vi "仪器连通测试VI.vi"(4 "断开通讯":bool, 7 "motor link":bool, 8 "error in (no error)":errorcluster caption="错误输入（无错误）", 9 "rotation num":dbl, 10 "target position":dbl=0.2 min=0.2 max=25.0 step=0.002) -> (0 "error out":errorcluster caption="错误输出", 1 "rotaion":dbl, 2 "position":dbl)   [LabVIEW 2017]
doc: "该模板用于创建子VI。"
uses:
  motor control.ctl
panel:
  in  "DaisyChain settings for rotation":T1={"Register DC"=FALSE, "DaisyChain Search?"=TRUE, "Device ID"=1}
  in  "USB settings for rotation":cluster{"S/N":string, "USB Search?":bool}={"S/N"="0135500392", "USB Search?"=FALSE}
  in  "System no. 2":i32=1 min=1 step=1
  in  "DaisyChain setting for move":T1={"Register DC"=FALSE, "DaisyChain Search?"=TRUE, "Device ID"=1}
  in  "USB setting for move":cluster{"S/N":string, "USB Search?":bool}={"S/N"="0135500392", "USB Search?"=FALSE}
  in  "minimal rot error":dbl=0.001
  in  "minimal error":dbl=0.001
  in  "motor control":T2={"System no."=1, "Conn. \nAxes"=[], "当前数值"=[]} {"System no." min=1 step=1}
  in  "System no.":i32=1 min=1 step=1
  # "parameter set"
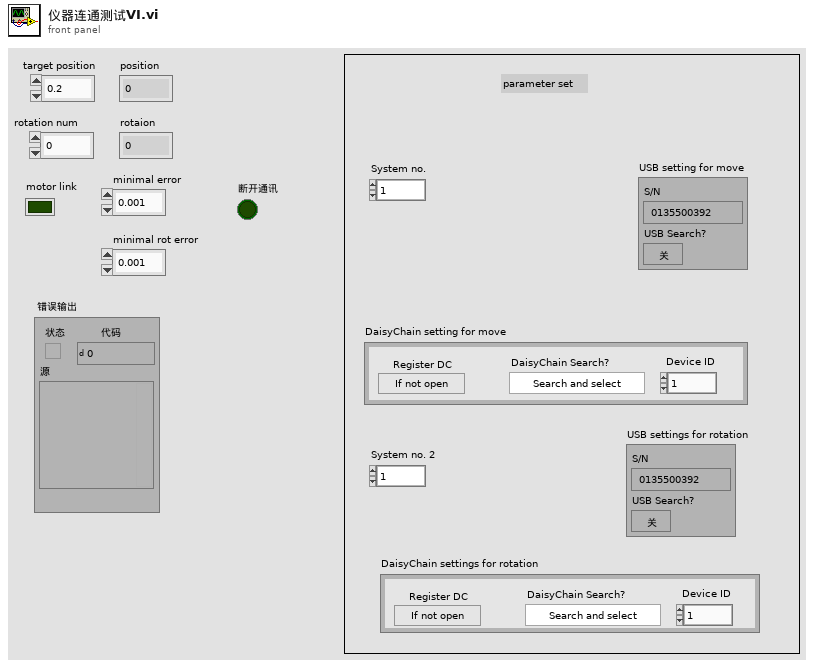
[diagram p1: front panel]
types:
  T1 = cluster{"Register DC":bool, "DaisyChain Search?":bool, "Device ID":i32}
  T2 = typedef "motor control.ctl" = cluster{"System no.":i32, "Conn. \nAxes":string[], "当前数值":dbl[]}
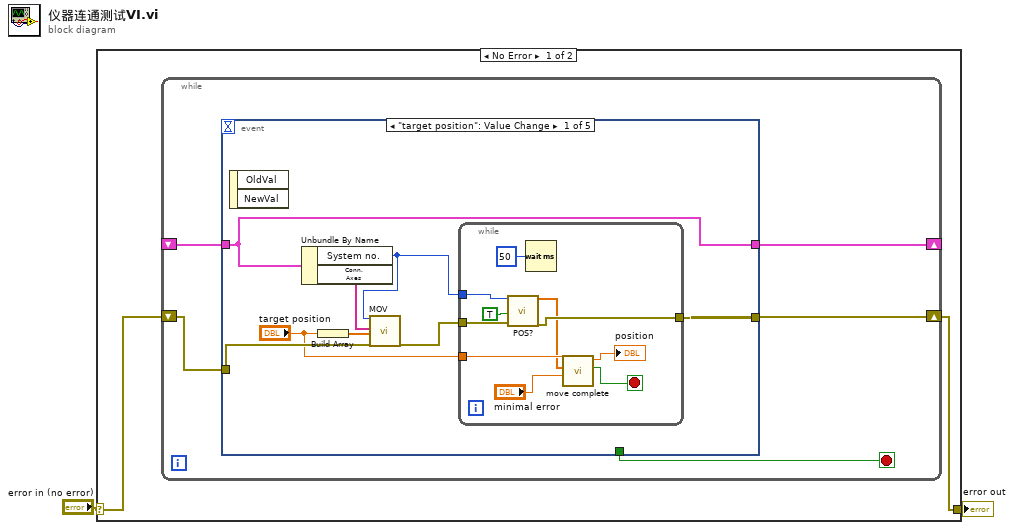
[diagram p0: block diagram]
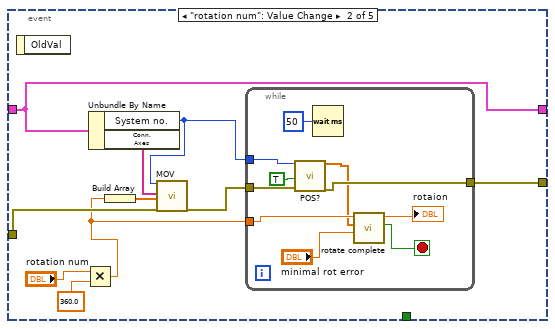
[diagram p2: hidden frame]
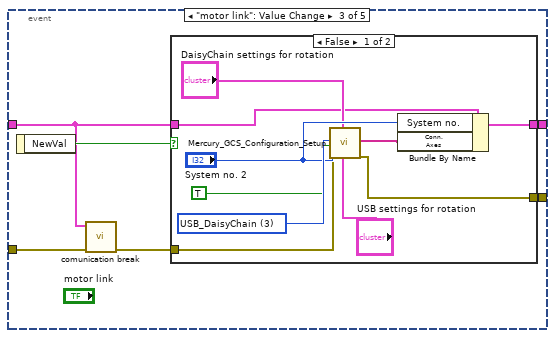
[diagram p3: hidden frame]
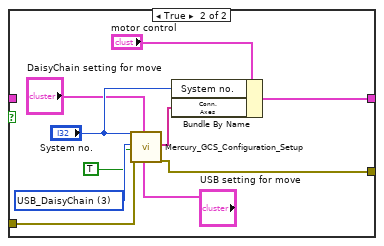
[diagram p4: hidden frame]
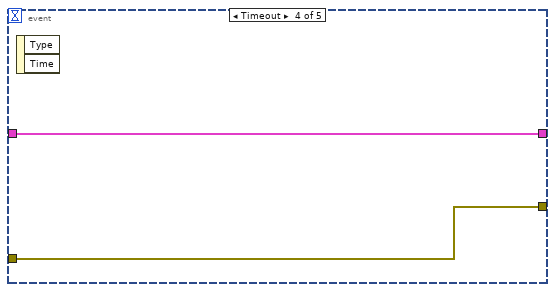
[diagram p5: hidden frame]
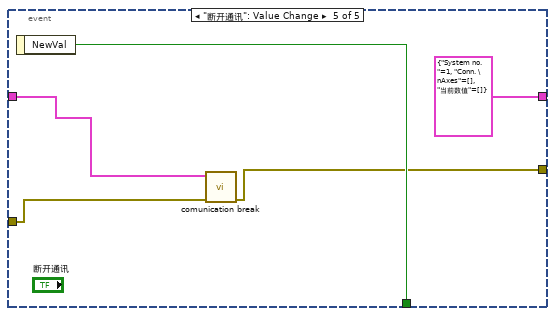
[diagram p6: hidden frame]
diagram:
  n1 = case shown="No Error" "error in (no error)" {
    selector: "error in (no error)" -> [w3 w81]
    tunnel: [w4 w81] -> w1
    frame No Error {
      n2 = while {
        shift-right: [w6] -> w4
        shift-left: w3 -> [w7]
        shift-right: [w9] -> _
        shift-left: _ -> [w8]
        stop <- w5 stop-if-true
        n3 = event shown="[0] \"target position\": Value Change" {
          selector: _ -> [_ _ _ _ _]
          dyn-events: _ -> [_ _ _ _ _]
          timeout: _ -> [_ _ _ _ _]
          tunnel: [w11 w31 w53 w74 w77] -> w6
          tunnel: w7 -> [w16 w36 w50 w74 w78]
          tunnel: [w15 w35 w52 w75 T2 {"System no."=1, "Conn. \nAxes"=[], "当前数值"=[]} ("motor control 2")] -> w9
          tunnel: w8 -> [w15 w35 w48 w75 w79]
          tunnel: [_ _ _ _ w80] -> w5
          event "target position": Value Change {
            n4 = event-data() -> ()  [unwired: 1 in, 2 out]
            n5 = Unbundle By Name(w15) -> ("System no."=w14:i32, "Conn. \nAxes"=w17:string[])
            n6 = Build Array("target position") -> (w12:dbl[])
            n7 = call "MOV.vi"("System no."=w14, "Axes to move"=w17, "Position values"=w12, "error in"=w16) -> ("error out"=w13:errorcluster)  [unwired: 15 in]
            n8 = while {
              tunnel: w14 -> [w27]
              tunnel: w13 -> [w25]
              tunnel: [w24] -> w11
              tunnel: "target position" -> [w21]
              stop <- w18 stop-if-true
              n9 = call "POS?.vi"("System no."=w27, "All axes?"=TRUE, "error in"=w25) -> ("Position"=w20:dbl[], "error out"=w24:errorcluster)  [unwired: 15 in]
              n10 = Wait (ms)(milliseconds to wait=u32 50 ("等待时间（毫秒）")) -> ()  [unwired: 1 out]
              n11 = call "move complete.vi"("minimal error"="minimal error", "Position"=w20, "target position"=w21) -> (2:w18:bool, "position output"=→"position":dbl)  [unwired: 6 in, 1 out]
            }
          }
          event "rotation num": Value Change {
            n12 = event-data() -> ()  [unwired: 1 in, 1 out]
            n13 = Multiply(x="rotation num", y=360.0) -> (x*y=w28:dbl)
            n14 = Unbundle By Name(w35) -> ("System no."=w34:i32, "Conn. \nAxes"=w37:string[])
            n15 = Build Array(w28) -> (w32:dbl[])
            n16 = call "MOV.vi"("System no."=w34, "Axes to move"=w37, "Position values"=w32, "error in"=w36) -> ("error out"=w33:errorcluster)  [unwired: 15 in]
            n17 = while {
              tunnel: w34 -> [w47]
              tunnel: w33 -> [w45]
              tunnel: [w44] -> w31
              tunnel: w28 -> [w42]
              stop <- w39 stop-if-true
              n18 = call "POS?.vi"("System no."=w47, "All axes?"=TRUE, "error in"=w45) -> ("Position"=w41:dbl[], "error out"=w44:errorcluster)  [unwired: 15 in]
              n19 = Wait (ms)(milliseconds to wait=u32 50 ("等待时间（毫秒）")) -> ()  [unwired: 1 out]
              n20 = call "rotate complete.vi"("minimal error"="minimal rot error", "current rotation"=w41, "target rotation"=w42) -> ("rot complete"=w39:bool, "rotation number"=→"rotaion":dbl)  [unwired: 6 in, 1 out]
            }
          }
          event "motor link": Value Change {
            n21 = event-data() -> ("NewVal"=w51:bool)  [unwired: 1 in]
            n22 = call "comunication break.vi"("错误输入（无错误）"=w50, "motor control输入"=w48) -> ("错误输出"=w49:errorcluster)  [unwired: 9 in]
            n23 = case shown="False" w51 {
              tunnel: w49 -> [w56 w71]
              tunnel: [w55 w70] -> w53
              tunnel: [w57 w66] -> w52
              tunnel: w48 -> [w54 _]
              frame False {
                w63 = u16 3 items=["RS232", "RS232 DaisyChain", "USB", "USB_DaisyChain"] ("Interface")
                n24 = call "Mercury_GCS_Configuration_Setup.vi"("System no."="System no. 2", "Interface"=w63, "All axes?"=TRUE ("Switch servo on?"), "error in"=w56, "DaisyChain settings"="DaisyChain settings for rotation", "USB settings"="USB settings for rotation") -> ("Conn. \nAxes"=w60:string[], "error out"=w55:errorcluster)  [unwired: 7 in, 5 out]
                n25 = Bundle By Name(cluster=w54, "System no."="System no. 2", "Conn. \nAxes"=w60) -> (w57:T2)
              }
              frame True {
                w73 = u16 3 items=["RS232", "RS232 DaisyChain", "USB", "USB_DaisyChain"] ("Interface")
                n26 = call "Mercury_GCS_Configuration_Setup.vi"("System no."="System no.", "Interface"=w73, "All axes?"=TRUE ("Switch servo on?"), "error in"=w71, "DaisyChain settings"="DaisyChain setting for move", "USB settings"="USB setting for move") -> ("Conn. \nAxes"=w67:string[], "error out"=w70:errorcluster)  [unwired: 7 in, 5 out]
                n27 = Bundle By Name(cluster="motor control", "System no."="System no.", "Conn. \nAxes"=w67) -> (w66:T2)
              }
            }
          }
          event Timeout {
            n28 = event-data() -> ()  [unwired: 1 in, 2 out]
          }
          event "断开通讯": Value Change {
            n29 = event-data() -> ("NewVal"=w80:bool)  [unwired: 1 in]
            n30 = call "comunication break.vi"("错误输入（无错误）"=w78, "motor control输入"=w79) -> ("错误输出"=w77:errorcluster)  [unwired: 9 in]
          }
        }
      }
    }
    frame Error {
    }
  }
  "error out" <- w1
